vi "Write Alarm Limits - All.vi"(8 "error in (no error)":errorcluster, 10 "alarm limits":T1={"Active"=FALSE, "Low Alarm Limit"=0.0, "Low Warning Limit"=0.0, "High Warning Limit"=0.0, "High Alarm Limit"=0.0, "Low Alarm Severity"=enum."major", "Low Warning Severity"=enum."minor", "High Warning Severity "=enum."minor", "High Alarm Severity"=enum."major", "Hysteresis"=0.0}, 11 "NT Scalar (Numeric) in":refnum<class "NT Scalar (Numeric).lvclass">) -> (0 "error out":errorcluster, 3 "NT Scalar (Numeric) out":refnum<class "NT Scalar (Numeric).lvclass">)   [LabVIEW 2020, in "PV Access.lvlib" / "PV Data.lvlib" / "NT Scalar (Numeric).lvclass"]
uses:
  NT Scalar (Numeric).lvclass
  NT Scalar (Numeric).lvclass/NT Scalar (Numeric).ctl
  Alarm Severity.ctl
  PV Data.lvlib
  Alarm Limits.ctl
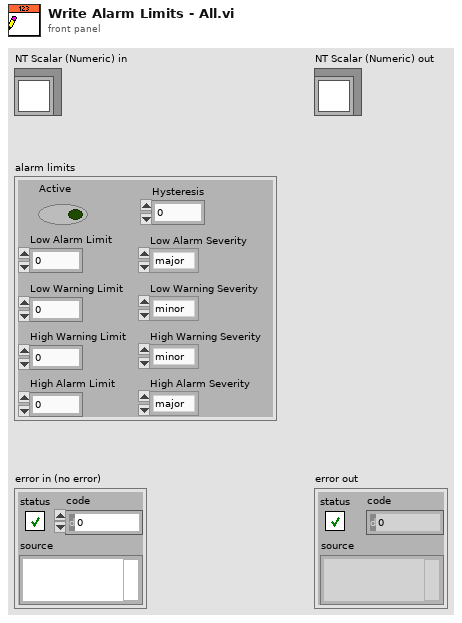
[diagram p1: front panel]
types:
  T1 = typedef "PV Access.lvlib/PV Data.lvlib/Alarm Limits.ctl" = cluster{"Active":bool, "Low Alarm Limit":dbl, "Low Warning Limit":dbl, "High Warning Limit":dbl, "High Alarm Limit":dbl, "Low Alarm Severity":T2, "Low Warning Severity":T2, "High Warning Severity ":T2, "High Alarm Severity":T2, "Hysteresis":dbl}
  T2 = typedef "PV Access.lvlib/PV Data.lvlib/Alarm Severity.ctl" = enum32{"no", "minor", "major", "record", "invalid", "undefined"}
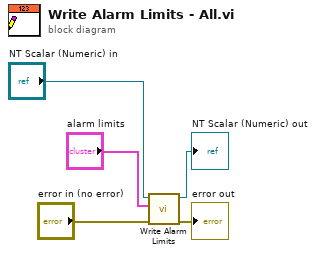
[diagram p0: block diagram]
diagram:
  n1 = call-dynamic "Write Alarm Limits.vi"("error in"="error in (no error)", "alarm limits"="alarm limits", "Has Alarm Limits in"="NT Scalar (Numeric) in") -> ("error out"=→"error out":errorcluster, "Has Alarm Limits out"=→"NT Scalar (Numeric) out":refnum<class "NT Scalar (Numeric).lvclass">)  [unwired: 7 in]
